vi "RT Main.vi"() -> ()   [LabVIEW 2016]
panel:
  out "error IO":errorcluster
  out "N Steps":u16[](array[numeric])
  out "Time":u32[](array[numeric])
  in  "Time per image (ms)":u32=1000
  in  "Number of Images":i32=10
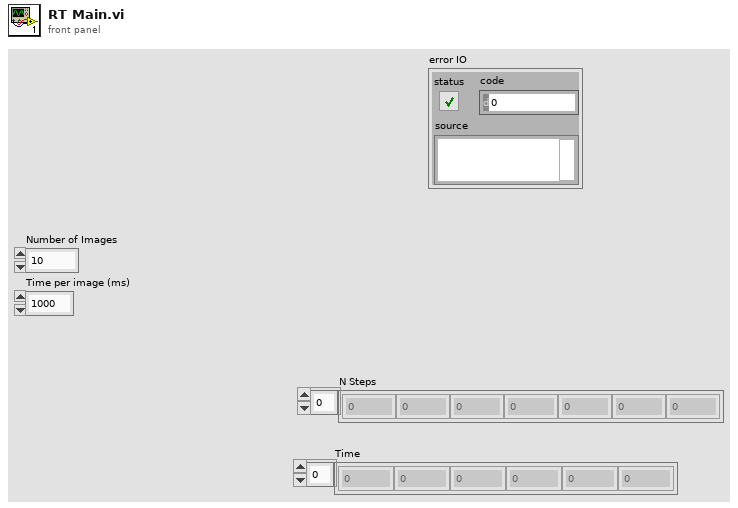
[diagram p1: front panel]
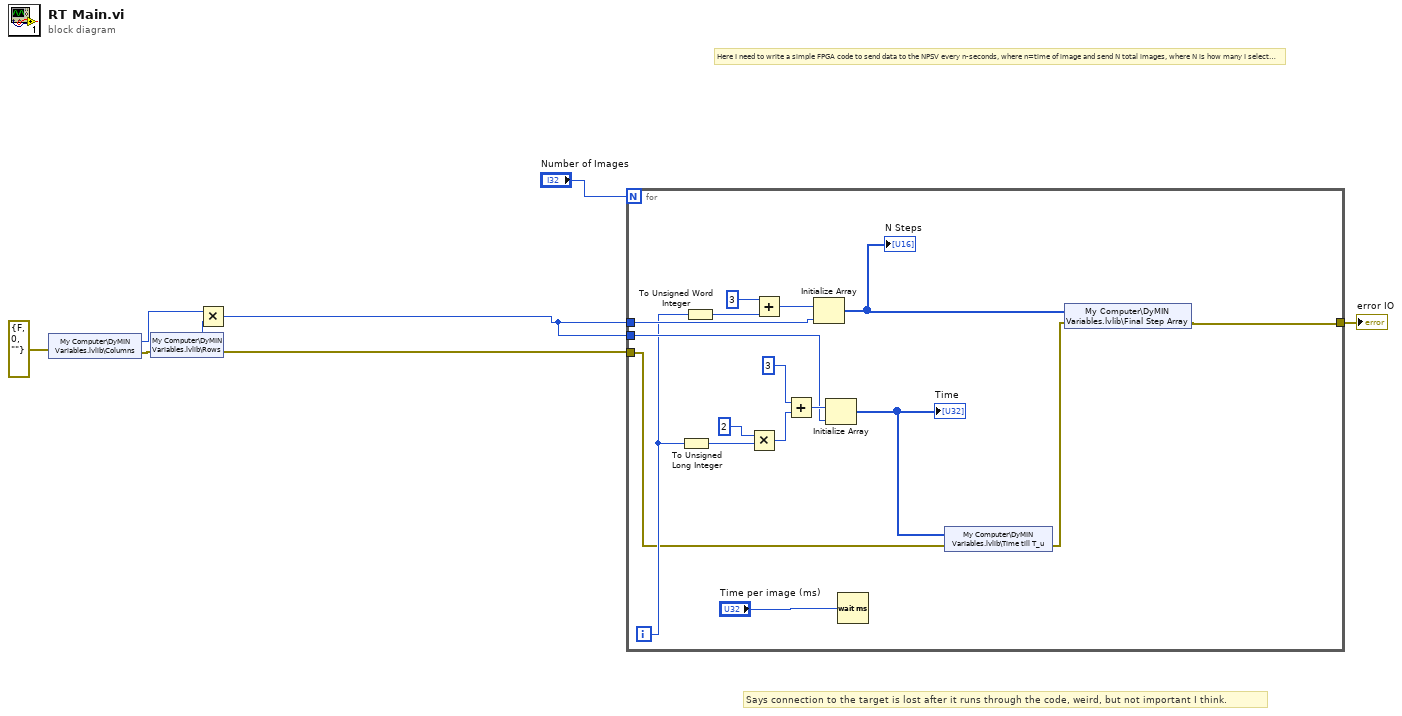
[diagram p0: block diagram]
diagram:
  # "Says connection to the target is lost after it runs through the code, weird, but not important I think."
  # "Here I need to write a simple FPGA code to send data to the NPSV every n-seconds, where n=time of image and send N total images, where N is how many I select from Slidebook."
  n1 = shared-variable "My Computer\\DyMIN Variables.lvlib\\Columns"(error in=errorcluster {"status"=FALSE, "code"=0, "source"=""} ("error in (no error)")) -> (w7:u16, error out=w5:errorcluster)
  n2 = shared-variable "My Computer\\DyMIN Variables.lvlib\\Rows"(error in=w5) -> (w6:u16, error out=w1:errorcluster)
  n3 = Multiply(x=w7, y=w6) -> (x*y=w2:u16)
  n4 = for {
    N: "Number of Images" -> [_]
    tunnel: w1 -> [w12]
    tunnel: w2 -> [w18]
    tunnel: w2 -> [w17]
    tunnel: [w9] -> w4
    i -> [w15]
    n5 = To Unsigned Long Integer(number=w15) -> (unsigned 32bit integer=w13:u32)
    n6 = To Unsigned Word Integer(number=w15) -> (unsigned 16bit integer=w14:u16)
    n7 = Multiply(x=u32 2, y=w13) -> (x*y=w23:u32)
    n8 = Add(x=u16 3, y=w14) -> (x+y=w20:u16)
    n9 = Add(x=u32 3, y=w23) -> (x+y=w19:u32)
    n10 = Initialize Array(w20, w18) -> (w16:u16[])
    "N Steps" <- w16
    n11 = Initialize Array(w19, w17) -> (w10:u32[])
    "Time" <- w10
    n12 = Wait (ms)(milliseconds to wait="Time per image (ms)") -> ()  [unwired: 1 out]
    n13 = shared-variable "My Computer\\DyMIN Variables.lvlib\\Time till T_u"(w10, error in=w12) -> (error out=w11:errorcluster)
    n14 = shared-variable "My Computer\\DyMIN Variables.lvlib\\Final Step Array"(w16, error in=w11) -> (error out=w9:errorcluster)
  }
  "error IO" <- w4
